vi "Sandbox.vi"   [LabVIEW 2017]
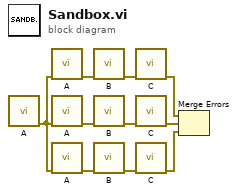
[diagram p0: block diagram]
diagram:
  n1 = call "A.vi"() -> ("error out"=w2:errorcluster)  [unwired: 11 in]
  n2 = call "A.vi"("A error in (no error)"=w2) -> ("error out"=w7:errorcluster)  [unwired: 10 in]
  n3 = call "A.vi"("A error in (no error)"=w2) -> ("error out"=w10:errorcluster)  [unwired: 10 in]
  n4 = call "A.vi"("A error in (no error)"=w2) -> ("error out"=w4:errorcluster)  [unwired: 10 in]
  n5 = call "B.vi"("error in (no error)"=w7) -> ("error out"=w8:errorcluster)  [unwired: 10 in]
  n6 = call "B.vi"("error in (no error)"=w10) -> ("error out"=w9:errorcluster)  [unwired: 10 in]
  n7 = call "B.vi"("error in (no error)"=w4) -> ("error out"=w3:errorcluster)  [unwired: 10 in]
  n8 = call "C.vi"("error in (no error)"=w8) -> ("C error out"=w6:errorcluster)  [unwired: 10 in]
  n9 = call "C.vi"("error in (no error)"=w9) -> ("C error out"=w5:errorcluster)  [unwired: 10 in]
  n10 = call "C.vi"("error in (no error)"=w3) -> ("C error out"=w1:errorcluster)  [unwired: 10 in]
  n11 = Merge Errors(w6, w5, w1) -> ()  [unwired: 1 out]
